vi "Get cluster section.vi"(8 "error in (no error)":errorcluster, 9 "Name (none)":string, 10 "Array Positions (none)":i32[](array[numeric]), 11 "Data in":T2 {"Device Ref" format="%.0x"; "Section Ref" format="%.0x"}) -> (0 "error out":errorcluster, 1 "Section Ptr":T1=18446744073709551615 format="%.0x", 2 "Name":string, 3 "Data out":T2 {"Device Ref" format="%.0x"; "Section Ref" format="%.0x"})   [LabVIEW 2016, in "DCM System Explorer.lvlib"]
uses:
  DCM System Explorer.lvlib
  <vilib>/NI Veristand/Custom Device API/Custom Device Item Ref.ctl
  <vilib>/NI VeriStand/Custom Device API/Custom Device API.lvlib
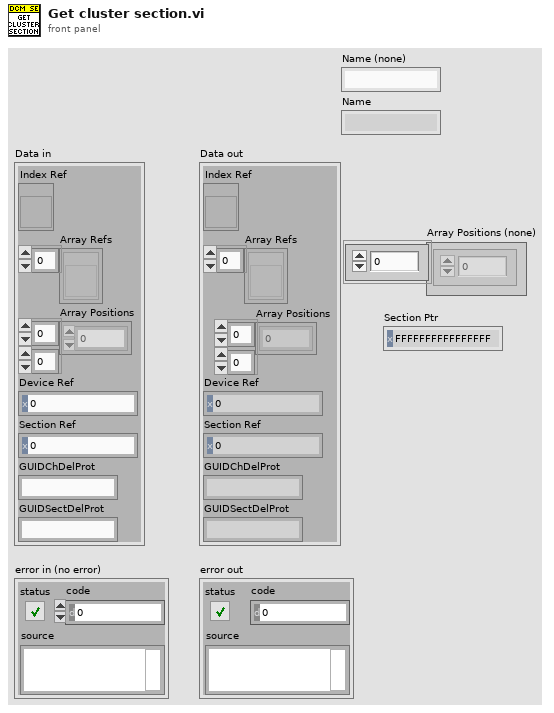
[diagram p1: front panel]
types:
  T1 = typedef "Custom Device API.lvlib/Custom Device Item Ref.ctl" = u64
  T2 = cluster{"Index Ref":refnum<vi>, "Array Refs":refnum<vi>[], "Array Positions":i32[][], "Device Ref":T1, "Section Ref":T1, "GUIDChDelProt":string, "GUIDSectDelProt":string}
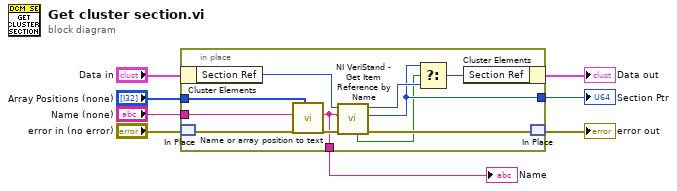
[diagram p0: block diagram]
diagram:
  n1 = in-place {
    in-place-border: "Array Positions (none)" -> [w15]
    in-place-border: [w11] -> w3
    in-place-border: "Name (none)" -> [w14]
    in-place-border: [w9] -> w1
    n2 = in-place-cluster #1("Data in") -> ("Section Ref"=w18:T1)
    n3 = in-place-match #2("error in (no error)") -> (w17:errorcluster)
    n4 = call "Name or array position to text.vi"("Array Positions (none)"=w15, "Name in"=w14) -> ("Name out"=w9:string)  [unwired: 9 in]
    n5 = call <vilib>:"NI VeriStand - Get Item Reference by Name.vi"("error in (no error)"=w17, "Item Name"=w9, "Parent Ref in"=w18) -> ("error out"=w16:errorcluster, "Item Ref"=w11:T1, "Parent Ref out"=w12:T1, "Found"=w10:bool)  [unwired: 5 in]
    n6 = Select(t=w11, s=w10, f=w12) -> (s? t:f=w13:T1)
    n7 = in-place-cluster #1("Section Ref"=w13) -> (→"Data out":T2)
    n8 = in-place-match #2(w16) -> (→"error out":errorcluster)
  }
  "Section Ptr" <- w3
  "Name" <- w1
